vi "WaitOnEventSync.vi"(8 "error in (no error)":errorcluster, 11 "ModuleAdmin":refnum<class "ModuleAdmin.lvclass">) -> (0 "error out":errorcluster, 3 "ModuleAdmin":refnum<class "ModuleAdmin.lvclass">)   [LabVIEW 2018, in "ModuleAdmin.lvlib" / "ModuleAdmin.lvclass"]
uses:
  ModuleAdmin.lvclass
  <vilib>/Utility/error.llb/Error Cluster From Error Code.vi
  <vilib>/ErrorRing/Error Ring.xnode
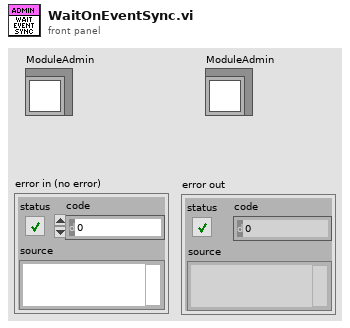
[diagram p1: front panel]
types:
  T1 = typedef "Rendezvous RefNum" = refnum<k1>
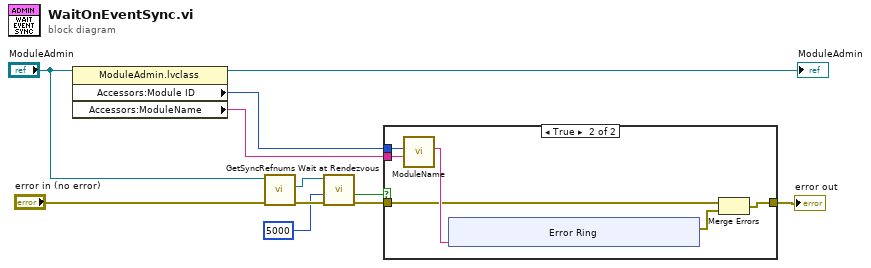
[diagram p0: block diagram]
diagram:
  n1 = property class="ModuleAdmin.lvclass"(reference="ModuleAdmin") -> (reference out=→"ModuleAdmin":refnum<class "ModuleAdmin.lvclass">, "Accessors:Module ID"=w4:i32, "Accessors:ModuleName"=w2:string)  [unwired: 1 in, 1 out]
  n2 = call "GetSyncRefnums.vi"("error in (no error)"="error in (no error)", "ModuleAdmin"="ModuleAdmin") -> ("error out"=w10:errorcluster, "rndzv_EventSync"=w5:T1)  [unwired: 6 in, 2 out]
  n3 = call <vilib>:"Wait at Rendezvous.vi"("error in (no error)"=w10, "ms timeout (-1)"=5000, "rendezvous"=w5) -> ("error out"=w7:errorcluster, "timed out"=w8:bool)  [unwired: 2 in, 1 out]
  n4 = case shown="True" w8 {
    tunnel: w7 -> [w12 w14]
    tunnel: [w12 w13] -> w6
    tunnel: w4 -> [_ w18]
    tunnel: w2 -> [_ w17]
    frame False {
    }
    frame True {
      n5 = call "ModuleName.vi"("Name"=w17, "ModuleID"=w18) -> ("ModuleName"=w16:string)  [unwired: 9 in]
      n6 = xnode "Error Ring"("parameter 0"=w16) -> ("error out"=w15:errorcluster)
      n7 = Merge Errors(w14, w15) -> (w13:errorcluster)
    }
  }
  "error out" <- w6
